vi "Confidence Intervals from PDF_PN.vi"(2 "Desired confidence interval (%)":dbl, 3 "PDF bin width":dbl, 4 "Marginal 1D PDF":dbl[](array[numeric])) -> (0 "Lower limit scale factor on SD or SE":dbl, 1 "Upper limit scale factor on SD or SE":dbl)   [LabVIEW 2016]
panel:
  in  "Show graphics":bool
  out "PDF with CI markers":cluster{dbl[], "Marginal 1D PDF":dbl[]}[](graph)
  # "IMPORTANT!\nPDF must be normalised such that Sum(PDF(x)) * dx = 1"
  # "Paul Nathan\n06/12/2016"
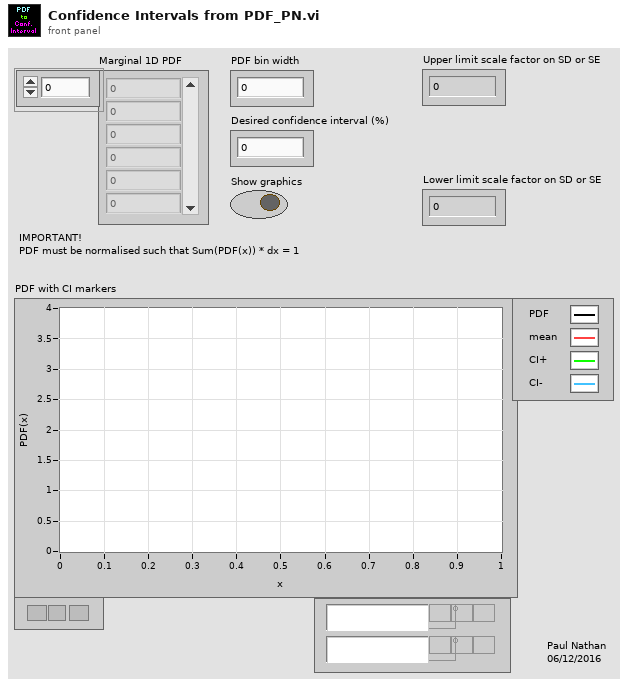
[diagram p1: front panel]
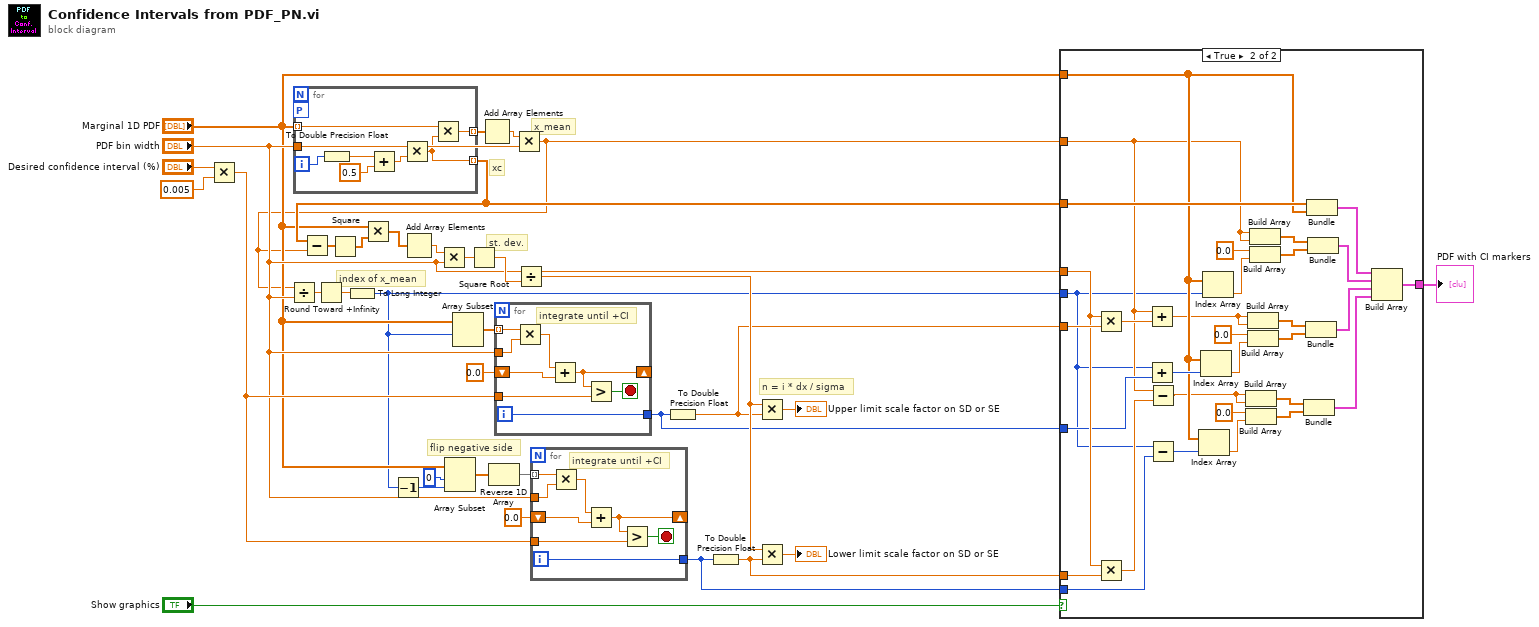
[diagram p0: block diagram]
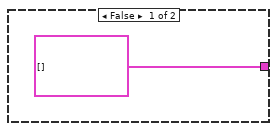
[diagram p2: hidden frame]
diagram:
  # "flip negative side"
  # "n = i * dx / sigma"
  # "index of x_mean"
  # "xc"
  # "st. dev."
  # "x_mean"
  n1 = Multiply(x="Desired confidence interval (%)", y=0.005) -> (x*y=w18:dbl)
  n2 = for {
    tunnel: "Marginal 1D PDF" -> [w39] mode=indexing
    tunnel: "PDF bin width" -> [w40]
    tunnel: [w38] -> w32 mode=indexing
    workers-P: _ -> [_]
    tunnel: [w37] -> w12 mode=indexing
    i -> [w42]
    n3 = To Double Precision Float(number=w42) -> (double precision float=w41:dbl)
    n4 = Add(x=w41, y=0.5) -> (x+y=w36:dbl)
    n5 = Multiply(x=w40, y=w36) -> (x*y=w37:dbl)
    n6 = Multiply(x=w39, y=w37) -> (x*y=w38:dbl)
  }
  n7 = Add Array Elements(numeric array=w32) -> (sum=w31:dbl)
  n8 = Multiply(x=w31, y="PDF bin width") -> (x*y=w6:dbl)
  n9 = Divide(x=w6, y="PDF bin width") -> (x/y=w27:dbl)
  n10 = Subtract(x=w12, y=w6) -> (x-y=w25:dbl[])
  n11 = Round Toward +Infinity(x=w27) -> (ceil(x): smallest int >= x=w28:dbl)
  n12 = Square(x=w25) -> (x^2=w26:dbl[])
  n13 = To Long Integer(number=w28) -> (32bit integer=w3:i32)
  n14 = Multiply(x="Marginal 1D PDF", y=w26) -> (x*y=w24:dbl[])
  n15 = Decrement(x=w3) -> (x-1=w4:i32)
  n16 = Add Array Elements(numeric array=w24) -> (sum=w30:dbl)
  n17 = Multiply(x=w30, y="PDF bin width") -> (x*y=w29:dbl)
  n18 = Array Subset(array="Marginal 1D PDF", index=0, length=w4) -> (w21:dbl[])
  n19 = Array Subset(array="Marginal 1D PDF", index=w3) -> (w23:dbl[])  [unwired: 1 in]
  n20 = Square Root(x=w29) -> (sqrt(x)=w16:dbl)
  n21 = Reverse 1D Array(array=w21) -> (reversed array=w20:dbl[])
  n22 = for {
    tunnel: w23 -> [w50] mode=indexing
    tunnel: "PDF bin width" -> [w49]
    tunnel: w18 -> [w45]
    shift-right: [w46] -> _
    shift-left: 0.0 ("y") -> [w48]
    tunnel: [w43] -> w8
    i -> [w43]
    stop <- w44 stop-if-true
    # "integrate until +CI"
    n23 = Multiply(x=w50, y=w49) -> (x*y=w47:dbl)
    n24 = Add(x=w47, y=w48) -> (x+y=w46:dbl)
    n25 = Greater?(x=w46, y=w45) -> (0:w44:bool)
  }
  n26 = Divide(x="PDF bin width", y=w16) -> (x/y=w15:dbl)
  n27 = for {
    tunnel: w20 -> [w58] mode=indexing
    tunnel: "PDF bin width" -> [w57]
    tunnel: w18 -> [w53]
    shift-right: [w54] -> _
    shift-left: 0.0 ("y") -> [w56]
    tunnel: [w51] -> w5
    i -> [w51]
    stop <- w52 stop-if-true
    # "integrate until +CI"
    n28 = Multiply(x=w58, y=w57) -> (x*y=w55:dbl)
    n29 = Add(x=w55, y=w56) -> (x+y=w54:dbl)
    n30 = Greater?(x=w54, y=w53) -> (0:w52:bool)
  }
  n31 = To Double Precision Float(number=w8) -> (double precision float=w11:dbl)
  n32 = To Double Precision Float(number=w5) -> (double precision float=w10:dbl)
  n33 = Multiply(x=w15, y=w11) -> (x*y=→"Upper limit scale factor on SD or SE":dbl)
  n34 = Multiply(x=w15, y=w10) -> (x*y=→"Lower limit scale factor on SD or SE":dbl)
  n35 = case shown="True" "Show graphics" {
    tunnel: w12 -> [_ w90]
    tunnel: w11 -> [_ w80]
    tunnel: w10 -> [_ w78]
    tunnel: "PDF bin width" -> [_ w77]
    tunnel: w8 -> [_ w76]
    tunnel: "Marginal 1D PDF" -> [_ w69]
    tunnel: w6 -> [_ w68]
    tunnel: w5 -> [_ w63]
    tunnel: w3 -> [_ w61]
    tunnel: [cluster{dbl[], "Marginal 1D PDF":dbl[]}[] [] w60] -> w2
    frame False {
    }
    frame True {
      n36 = Multiply(x=w77, y=w80) -> (x*y=w79:dbl)
      n37 = Multiply(x=w77, y=w78) -> (x*y=w67:dbl)
      n38 = Add(x=w68, y=w79) -> (x+y=w66:dbl)
      n39 = Add(x=w61, y=w76) -> (x+y=w75:i32)
      n40 = Subtract(x=w68, y=w67) -> (x-y=w65:dbl)
      n41 = Subtract(x=w61, y=w63) -> (x-y=w62:i32)
      n42 = Index Array(array=w69, index=w62) -> (element=w70:dbl)
      n43 = Index Array(array=w69, index=w75) -> (element=w84:dbl)
      n44 = Index Array(array=w69, index=w61) -> (element=w85:dbl)
      n45 = Build Array(w65, w65) -> (w73:dbl[])
      n46 = Build Array(0.0 ("y"), w70) -> (w71:dbl[])
      n47 = Build Array(w66, w66) -> (w81:dbl[])
      n48 = Build Array(0.0 ("y"), w84) -> (w83:dbl[])
      n49 = Build Array(w68, w68) -> (w89:dbl[])
      n50 = Build Array(0.0 ("y"), w85) -> (w87:dbl[])
      n51 = Bundle(w73, w71) -> (w64:cluster{dbl[], dbl[]})  [unwired: 1 out]
      n52 = Bundle(w81, w83) -> (w74:cluster{dbl[], dbl[]})  [unwired: 1 out]
      n53 = Bundle(w90, "Marginal 1D PDF"=w69) -> (w91:cluster{dbl[], "Marginal 1D PDF":dbl[]})  [unwired: 1 out]
      n54 = Bundle(w89, w87) -> (w86:cluster{dbl[], dbl[]})  [unwired: 1 out]
      n55 = Build Array(w91, w86, w74, w64) -> (w60:cluster{dbl[], "Marginal 1D PDF":dbl[]}[])
    }
  }
  "PDF with CI markers" <- w2
